vi "ButtonsEvent.vi"() -> ()   [LabVIEW 2023]
panel:
  in  "Stop Button":bool
  out "Boolean":bool
  in  "Play Button 2":bool
  in  "Play Button":bool
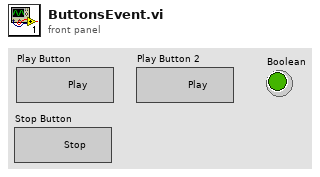
[diagram p1: front panel]
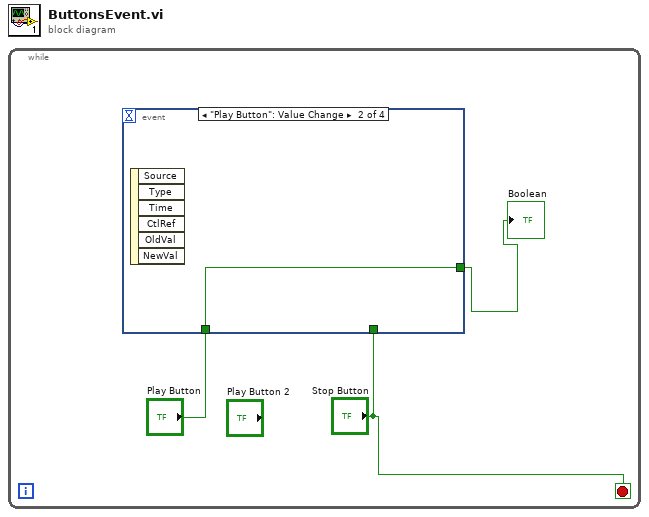
[diagram p0: block diagram]
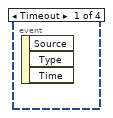
[diagram p2: hidden frame]
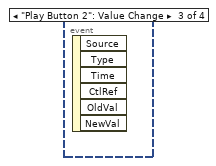
[diagram p3: hidden frame]
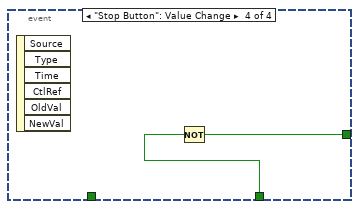
[diagram p4: hidden frame]
diagram:
  n1 = while {
    stop <- "Stop Button" stop-if-true
    n2 = event shown="[1] \"Play Button\": Value Change" {
      selector: _ -> [_ _ _ _]
      dyn-events: _ -> [_ _ _ _]
      timeout: _ -> [_ _ _ _]
      tunnel: "Stop Button" -> [_ _ _ w6]
      tunnel: [_ w4 _ w5] -> w2
      tunnel: "Play Button" -> [_ w4 _ _]
      event Timeout {
        n3 = event-data() -> ()  [unwired: 1 in, 3 out]
      }
      event "Play Button": Value Change {
        n4 = event-data() -> ()  [unwired: 1 in, 6 out]
      }
      event "Play Button 2": Value Change {
        n5 = event-data() -> ()  [unwired: 1 in, 6 out]
      }
      event "Stop Button": Value Change {
        n6 = event-data() -> ()  [unwired: 1 in, 6 out]
        n7 = Not(x=w6) -> (.not. x?=w5:bool)
      }
    }
    "Boolean" <- w2
  }
